vi "Single Tone Measurements.vi"() -> ()   [LabVIEW 2023]
doc: "Demonstrates the measurement of the frequency and amplitude of the input signal. This example gives you the ability to narrow the search to a particular frequency using the advanced search criteria."
uses:
  <vilib>/measure/matone.llb/Extract Single Tone Information.vi
  <vilib>/measure/NI_MAPro.lvlib
panel:
  out "Amplitude error (ppm)":dbl(knob) scale=0.0..10.0
  out "Frequency error (ppm)":dbl(knob) scale=0.0..10.0
  in  "Noise \"bitVolt\"":dbl(slide)=-14.89795918367347
  in  "export mode":u16(ring)=1 items=["none", "input signal", "detected signal", "residual signal"]
  in  "advanced search":T1={"approx freq. (optional)"=-1.0, "search (+/- % of Fsampl.)"=1.0}
  in  "Block size":i32=200
  out "Amplitude Result":dbl format="%_6g"
  out "Frequency Result":dbl
  out "Exported signal spectrum (dBV)":T2(graph)
  in  "second tone":bool
  in  "Stop":bool
  out "Exported time signal":waveform(dbl)(graph)
  in  "Amplitude (V)":dbl=1.0
  in  "Frequency (Hz)":dbl=8067.89
  in  "Fs (Hz)":dbl=51200.0
  # "Overview: Shows how to use the Extract Single Tone Information VI to measure the frequency and amplitude of a tone in a signal.\nRequirements: LabVIEW Full Development System\nInstructions: \n1. Run the VI. Note the accuracy of the Analysis Results.\n2. Enable the addition of an interfering tone by clicking second tone, and note that the second tone is now detected.\n3. Set the advanced search approx freq. value to 8000 Hz and note that the correct tone is extracted.\n4. Click Stop to stop the VI."
  # "Input Signal"
  # "Analysis Results"
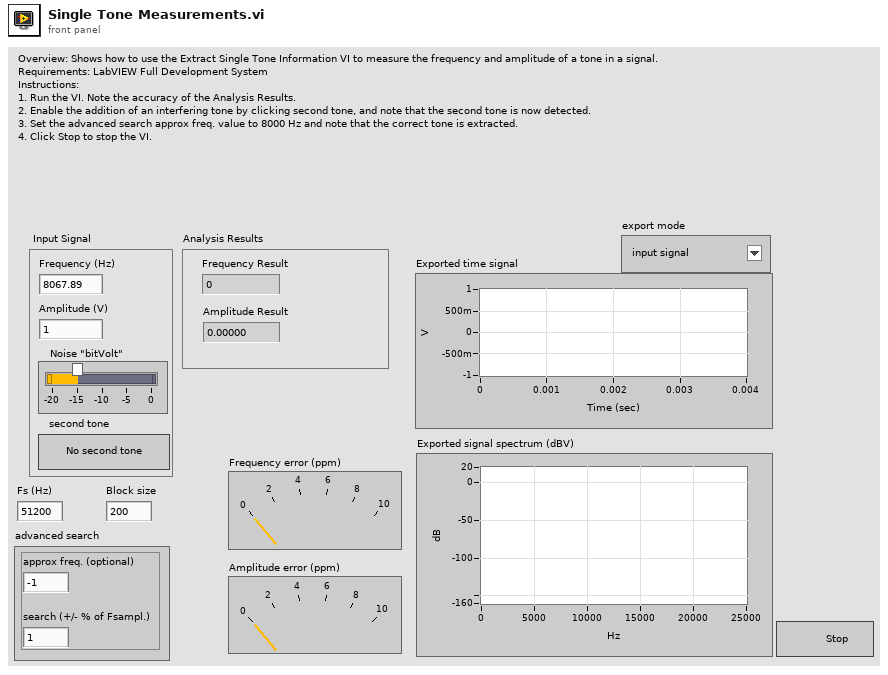
[diagram p1: front panel]
types:
  T1 = cluster{"approx freq. (optional)":dbl, "search (+/- % of Fsampl.)":dbl}
  T2 = cluster{"f0":dbl, "df":dbl, "dB Spectrum (Hann)":dbl[]}
  T3 = cluster{"exported time signal":waveform(dbl), "exported spectrum (dB)":cluster{"f0":dbl, "df":dbl, "dB Spectrum (Hann)":dbl[]}}
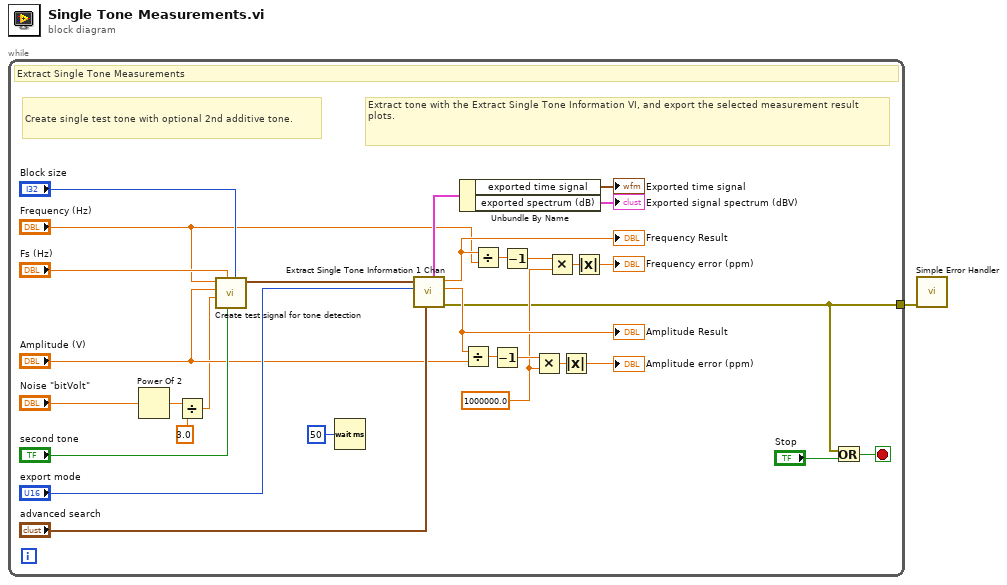
[diagram p0: block diagram]
diagram:
  n1 = while {
    tunnel: [w3] -> w1
    stop <- w4 stop-if-true
    w5 = 1000000.0
    # "Extract tone with the Extract Single Tone Information VI, and export the selected measurement result plots."
    # "Create single test tone with optional 2nd additive tone."
    # "Extract Single Tone Measurements"
    n2 = Power Of 2(x="Noise \"bitVolt\"") -> (2^x=w30:dbl)
    n3 = Divide(x=w30, y=3.0) -> (x/y=w7:dbl)
    n4 = call "Create test signal for tone detection.vi"("block size"="Block size", "second tone"="second tone", "sampling frequency (Hz)"="Fs (Hz)", "Noise level (Vrms)"=w7, "Tone amplitude"="Amplitude (V)", "Tone frequency (Hz)"="Frequency (Hz)") -> ("Test signal"=w19:waveform(dbl))  [unwired: 5 in]
    n5 = Wait (ms)(milliseconds to wait=u32 50) -> ()  [unwired: 1 out]
    n6 = call-poly <vilib>:"Extract Single Tone Information 1 Chan.vi"("advanced search"="advanced search", "export mode"="export mode", "time signal in"=w19) -> ("error out"=w3:errorcluster, "detected amplitude"=w20:dbl, "detected frequency"=w21:dbl, "exported signals"=w16:T3)  [unwired: 3 in, 2 out]
    "Frequency Result" <- w21
    "Amplitude Result" <- w20
    n7 = Unbundle By Name(w16) -> ("exported time signal"=→"Exported time signal":waveform(dbl), "exported spectrum (dB)"=→"Exported signal spectrum (dBV)":T2)
    n8 = Divide(x=w20, y="Amplitude (V)") -> (x/y=w24:dbl)
    n9 = Divide(x=w21, y="Frequency (Hz)") -> (x/y=w29:dbl)
    n10 = Decrement(x=w24) -> (x-1=w25:dbl)
    n11 = Decrement(x=w29) -> (x-1=w28:dbl)
    n12 = Multiply(x=w25, y=w5) -> (x*y=w26:dbl)
    n13 = Multiply(x=w28, y=w5) -> (x*y=w27:dbl)
    n14 = Absolute Value(x=w26) -> (abs(x)=→"Amplitude error (ppm)":dbl)
    n15 = Absolute Value(x=w27) -> (abs(x)=→"Frequency error (ppm)":dbl)
    n16 = Or(x=w3, y="Stop") -> (x .or. y?=w4:bool)
  }
  n17 = call <vilib>:"Simple Error Handler.vi"("error in (no error)"=w1) -> ()  [unwired: 4 in, 5 out]
